vi "Read connections status.vi"(8 "error in (no error)":errorcluster, 11 "TCP slave in":refnum<class "TCP Slave.lvclass">) -> (0 "error out":errorcluster, 2 "connections":T1(array[cluster]), 3 "TCP slave out":refnum<class "TCP Slave.lvclass">)   [LabVIEW 2018, in "SubVIs.lvlib" / "TCP Slave.lvclass"]
uses:
  TCP Slave.lvclass
  TCP Slave.lvclass/TCP Slave.ctl
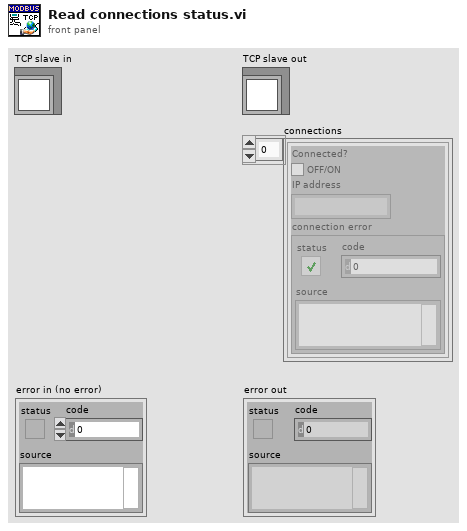
[diagram p1: front panel]
types:
  T1 = cluster{"Connected?":bool, "IP address":string, "connection error":errorcluster}[]
  T2 = typedef "SubVIs.lvlib/TCP Slave.lvclass/Connection Counter.ctl" = cluster{"Currently Connected":u32, "Connection Records":refnum<data-value>[]}
  T3 = cluster{"Connected?":bool, "IP address":string, "connection error":errorcluster}
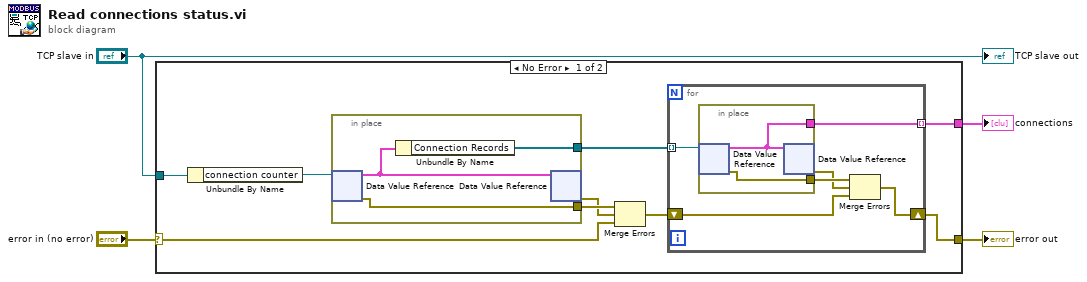
[diagram p0: block diagram]
diagram:
  n1 = case shown="No Error" "error in (no error)" {
    selector: "error in (no error)" -> [w6 w25]
    tunnel: "TCP slave in" -> [w13 _]
    tunnel: [w9 w25] -> w3
    tunnel: [w8 _] -> w2
    frame No Error {
      n2 = Unbundle By Name(w13) -> ("connection counter"=w12:refnum<data-value>)
      n3 = in-place {
        in-place-border: [w23] -> w11
        in-place-border: [w22] -> w7
        n4 = in-place-dvr #1(w12) -> (w24:T2, w22:errorcluster)
        n5 = Unbundle By Name(w24) -> ("Connection Records"=w23:refnum<data-value>[])
        n6 = in-place-dvr #1(w24) -> (w5:errorcluster)  [unwired: 1 out]
      }
      n7 = Merge Errors(w7, w5, w6) -> (w10:errorcluster)
      n8 = for {
        tunnel: w11 -> [w19] mode=indexing
        shift-right: [w18] -> w9
        shift-left: w10 -> [w14]
        tunnel: [w17] -> w8 mode=indexing
        n9 = in-place {
          in-place-border: [w21] -> w17
          in-place-border: [w20] -> w16
          n10 = in-place-dvr #2(w19) -> (w21:T3, w20:errorcluster)
          n11 = in-place-dvr #2(w21) -> (w15:errorcluster)  [unwired: 1 out]
        }
        n12 = Merge Errors(w16, w15, w14) -> (w18:errorcluster)
      }
    }
    frame Error {
    }
  }
  "error out" <- w3
  "connections" <- w2
  "TCP slave out" <- "TCP slave in"
